vi "Tosca-Tracking Thread.vi"(0 "IPC":T1) -> (15 "error out":errorcluster)   [LabVIEW 2020]
uses:
  IPC VIs/Tosca-IPC.ctl
  Classes/Parameters/Parameters.lvclass
  Digital Input VIs/Tosca-DI Queue Data.ctl
  Digital Input VIs/Tosca-Input Event.ctl
  Digital Input VIs/Tosca-Input Criterion.ctl
  epl-vi-lib/Utility VIs/Type Defs/Logic State.ctl
  Typedefs/Tosca-Accumulator.ctl
  Typedefs/Tosca-State AODO.ctl
  Typedefs/Tosca-AO Runtime.ctl
  Typedefs/Tosca-DO Runtime.ctl
  epl-vi-lib/Signal Synthesis VIs/4th Generation/Classes/SignalManager/SignalManager.lvclass
  Typedefs/Tosca-Synapse Start Data.ctl
  IPC VIs/Tosca-Message.ctl
  IPC VIs/Tosca-Message Action.ctl
  Typedefs/Tosca-Thread Type.ctl
  Imaging VIs/Tosca-2P-Notifier Data.ctl
  Typedefs/Tosca-MATLAB Queue Data.ctl
  Visual Stim VIs/Tosca-Grating.ctl
  Visual Stim VIs/Tosca-Grating Type.ctl
  Typedefs/Tosca-File IO Notification.ctl
  epl-vi-lib/TCP VIs/TCP Params.ctl
  epl-vi-lib/TCP VIs/TCP Write.vi
  Tosca-Globals.vi
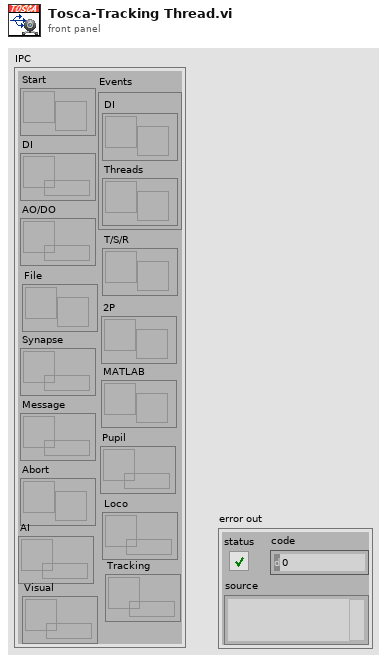
[diagram p1: front panel]
types:
  T1 = typedef "Tosca-IPC.ctl" = cluster{"Start":refnum<notifier>, "DI":refnum<queue>, "AO/DO":refnum<queue>, "Synapse":refnum<queue>, "Message":refnum<queue>, "Abort":refnum<notifier>, "Events":cluster{"DI":refnum<user-event>, "Threads ":refnum<user-event>}, "T/S/R":refnum<notifier>, "2P":refnum<notifier>, "MATLAB":refnum<notifier>, "Pupil":refnum<queue>, "Loco":refnum<queue>, "AI":refnum<queue>, "Tracking":refnum<queue>, "Visual":refnum<queue>, "File":refnum<notifier>}
  T2 = enum16{"big-endian, network order", "native, host order", "little-endian"}
  T3 = typedef "TCP Params.ctl" = cluster{"IP Address":string, "Port":i32}
  T4 = typedef "Tosca-Thread Type.ctl" = enum16{"None", "AODO", "Masker", "ET", "Imaging", "Pupil", "AI", "DI", "Camera", "TTL out", "Loco", "Visual"}
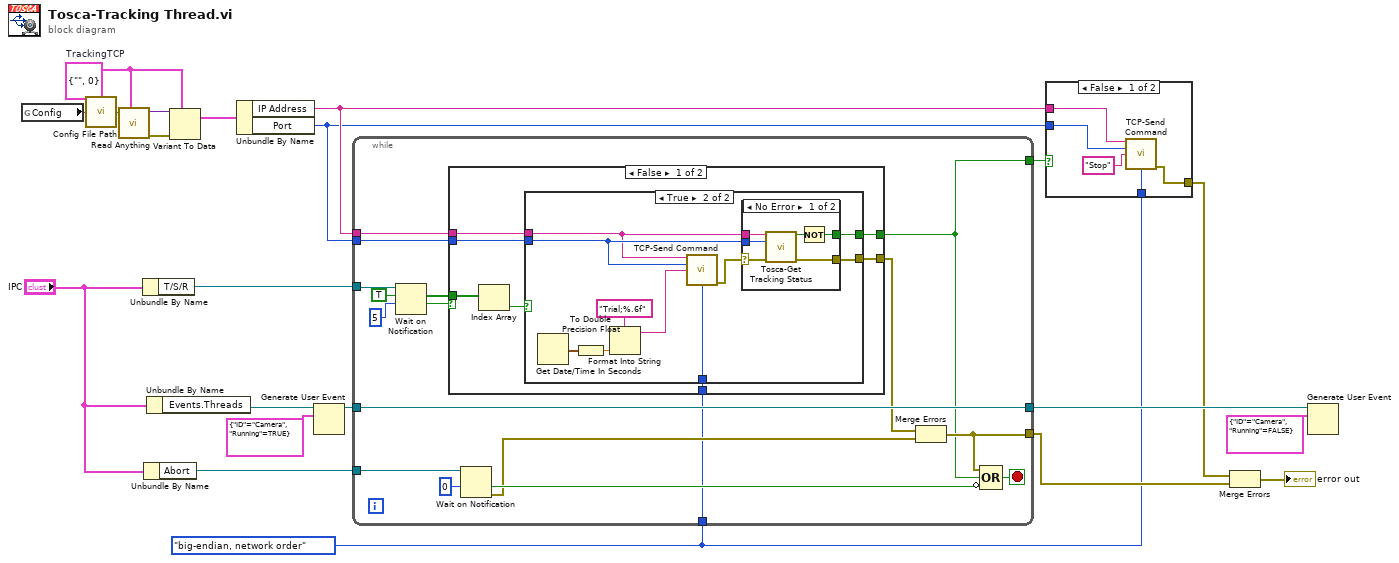
[diagram p0: block diagram]
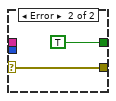
[diagram p3: hidden frame]
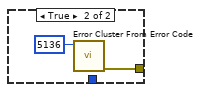
[diagram p5: hidden frame]
diagram:
  w1 = T2."big-endian, network order" ("byte order")
  w12 = T3 {"IP Address"="", "Port"=0}  # TrackingTCP
  n1 = global read "Tosca-Globals.vi" "Config"() -> (w2:string)
  n2 = call "Config File Path.vi"("AppName"=w2) -> ("Default config file name"=w11:path)
  n3 = call "Read Anything.vi"("Type of Anything"=w12, "Path (dialog)"=w11) -> ("Error Out"=w14:errorcluster, "Anything"=w13:variant)  [unwired: 7 in, 1 out]
  n4 = Unbundle By Name("IPC") -> ("T/S/R"=w3:refnum<notifier>)
  n5 = Unbundle By Name("IPC") -> ("Abort"=w16:refnum<notifier>)
  n6 = Unbundle By Name("IPC") -> ("Events.Threads"=w21:refnum<user-event>)
  n7 = Variant To Data(error in=w14, type=w12, Variant=w13) -> (data=w15:T3)  [unwired: 1 out]
  n8 = Unbundle By Name(w15) -> ("IP Address"=w6:string, "Port"=w5:i32)
  n9 = Generate User Event(user event=w21, event data cluster=cluster{"ID":T4, "Running":bool} {"ID"=enum."Camera", "Running"=TRUE} ("event data")) -> (user event out=w19:refnum<user-event>)  [unwired: 2 in, 1 out]
  n10 = while {
    tunnel: w19 -> [w38]
    tunnel: [w38] -> w18
    tunnel: w16 -> [w35]
    tunnel: w6 -> [w24]
    tunnel: w5 -> [w25]
    tunnel: [w31] -> w9
    tunnel: [w32] -> w8
    tunnel: w3 -> [w28]
    tunnel: w1 -> [w22]
    stop <- w34 stop-if-true
    n11 = Wait on Notification(notifier=w28, ignore previous (F)=TRUE, timeout in ms (-1)=5) -> (notification=w26:bool[], timed out?=w27:bool)  [unwired: 1 in, 2 out]
    n12 = case shown="False" w27 {
      tunnel: w26 -> [w44 _]
      tunnel: w24 -> [w43 _]
      tunnel: w25 -> [w42 _]
      tunnel: [w41 _] -> w23
      tunnel: [w40 _] -> w31
      tunnel: w22 -> [w39 _]
      frame False {
        n13 = Index Array(array=w44) -> (element=w45:bool)  [unwired: 1 in]
        n14 = case shown="True" w45 {
          tunnel: w43 -> [_ w49]
          tunnel: w42 -> [_ w50]
          tunnel: [_ w48] -> w41
          tunnel: [_ w47] -> w40
          tunnel: w39 -> [_ w46]
          frame False {
          }
          frame True {
            n15 = Get Date/Time In Seconds() -> (seconds since 1Jan1904=w53:timestamp)
            n16 = To Double Precision Float(number=w53) -> (double precision float=w52:dbl)
            n17 = Format Into String(format string="Trial;%.6f", w52) -> (resulting string=w54:string)  [unwired: 2 in, 1 out]
            n18 = call "TCP-Send Command.vi"("PXI Address"=w49, "Port"=w50, "Command"=w54, "byte order"=w46) -> ("error out"=w51:errorcluster)  [unwired: 11 in]
            n19 = case shown="No Error" w51 {
              selector: w51 -> [w61 w63]
              tunnel: w50 -> [w60 _]
              tunnel: w49 -> [w59 _]
              tunnel: [w58 w63] -> w48
              tunnel: [w56 TRUE ("Recording")] -> w47
              frame No Error {
                n20 = call "Tosca-Get Tracking Status.vi"("IP Address"=w59, "Port"=w60, "error in (no error)"=w61) -> ("Recording"=w57:bool, "error out"=w58:errorcluster)  [unwired: 11 in]
                n21 = Not(x=w57) -> (.not. x?=w56:bool)
              }
              frame Error {
              }
            }
          }
        }
      }
      frame True {
      }
    }
    n22 = Wait on Notification(notifier=w35, timeout in ms (-1)=0) -> (timed out?=w37:bool, error out=w33:errorcluster)  [unwired: 2 in, 2 out]
    n23 = Merge Errors(w23, w33) -> (w32:errorcluster)
    n24 = Compound Arithmetic op=OR(w32, w31, invert w37) -> (w34:bool)
  }
  n25 = case shown="False" w9 {
    tunnel: [w65 w69] -> w7
    tunnel: w6 -> [w67 _]
    tunnel: w5 -> [w66 _]
    tunnel: w1 -> [w64 _]
    frame False {
      n26 = call "TCP-Send Command.vi"("PXI Address"=w67, "Port"=w66, "Command"="Stop", "byte order"=w64) -> ("error out"=w65:errorcluster)  [unwired: 11 in]
    }
    frame True {
      n27 = call <vilib>:"Error Cluster From Error Code.vi"("error code (0)"=5136) -> ("error out"=w69:errorcluster)  [unwired: 8 in]
    }
  }
  n28 = Merge Errors(w7, w8) -> (→"error out":errorcluster)
  n29 = Generate User Event(user event=w18, event data cluster=cluster{"ID":T4, "Running":bool} {"ID"=enum."Camera", "Running"=FALSE} ("event data")) -> ()  [unwired: 2 in, 2 out]
